vi "muParser Demo2.vi"() -> ()   [LabVIEW 2015]
uses:
  muExpr/muExpr.lvclass/muExpr.ctl
  muExpr/Set Variable Values.vi
  muExpr/Eval.vi
  muExpr/Set Variable Value.vi
  mupLib/mupEval.vi
  mupLib/mupSetVarValue.vi
  mupLib/mupCheckError.vi
  <vilib>/Utility/error.llb/Error Cluster From Error Code.vi
  muExpr/muExpr.lvclass
panel:
  out "error out":errorcluster
  out "Result":dbl format="%#_13g"
  out "Variable Names":string[](array[string])
  in  "Expression":string="a*x+b"
  in  "varValues":dbl[](array[numeric])=[1.0, 1.0, 5.0] format="%#_13g"
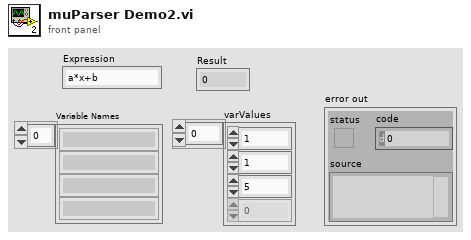
[diagram p1: front panel]
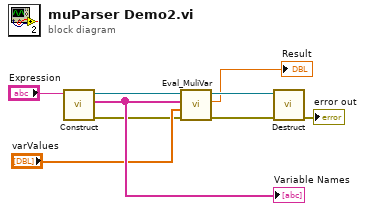
[diagram p0: block diagram]
diagram:
  n1 = call "Construct.vi"("Expression"="Expression") -> ("error out"=w4:errorcluster, "Variable Names"=w6:string[], "muExpr out"=w3:refnum<class "muExpr.lvclass">)  [unwired: 8 in]
  "Variable Names" <- w6
  n2 = call "Eval_MuliVar.vi"("error in (no error)"=w4, "varValues"="varValues", "varNames"=w6, "muExpr in"=w3) -> ("error out"=w7:errorcluster, "Result"=→"Result":dbl, "muExpr out"=w8:refnum<class "muExpr.lvclass">)  [unwired: 5 in]
  n3 = call "Destruct.vi"("error in (no error)"=w7, "muExpr in"=w8) -> ("error out"=→"error out":errorcluster)  [unwired: 9 in]
